vi "Decompose Cluster.vi"(8 "error in (no error)":errorcluster, 11 "Cluster":variant) -> (0 "error out":errorcluster, 3 "Cluster Elements":variant[](array[variant]))   [LabVIEW 2017, in "Composition.lvlib"]
doc: "Decomposes a cluster into its elements. The order of elements in the array follows the order of elements in the cluster."
uses:
  Composition.lvlib
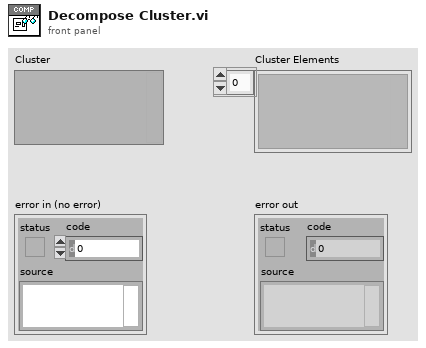
[diagram p1: front panel]
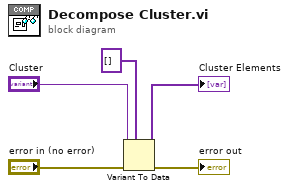
[diagram p0: block diagram]
diagram:
  n1 = Variant To Data(error in="error in (no error)", type=variant[] [], Variant="Cluster") -> (data=→"Cluster Elements":variant[], error out=→"error out":errorcluster)
